vi "decodeBaseRef.vi"(8 "error in (no error)":errorcluster, 10 "Base Reference":refnum<vi>, 11 "variant":variant) -> (0 "error out":errorcluster)   [LabVIEW 2015, in "MsgPack.lvlib"]
uses:
  MsgPack.lvlib
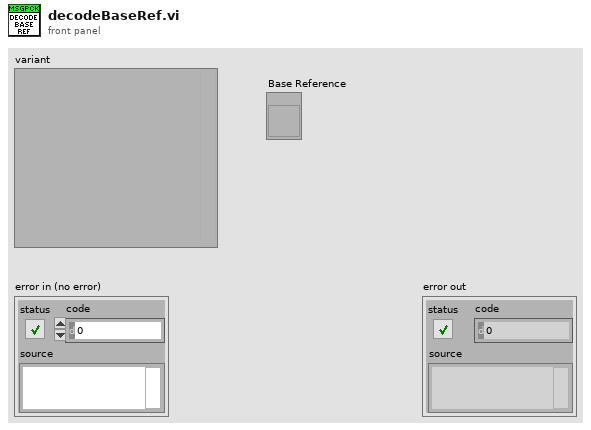
[diagram p1: front panel]
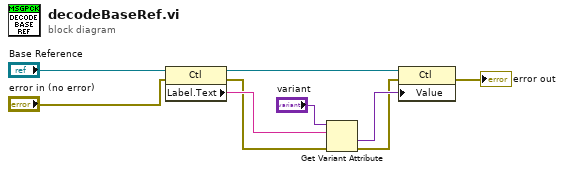
[diagram p0: block diagram]
diagram:
  n1 = property class="Ctl"(reference="Base Reference", error in="error in (no error)") -> (reference out=w4:refnum<vi>, error out=w5:errorcluster, "Label.Text"=w8:string)
  n2 = Get Variant Attribute(Variant="variant", name=w8, error in=w5) -> (value=w7:variant, error out=w6:errorcluster)  [unwired: 1 in, 2 out]
  n3 = property class="Ctl"(reference=w4, error in=w6, "Value"=w7) -> (error out=→"error out":errorcluster)  [unwired: 1 out]
